vi "Brute Force Dark Current Primary Logic Body.vi"(0 "Data Pin in":refnum<k21>, 1 "Barcodes in":string[](array[string]), 2 "Sync Pin in":refnum<k21>, 3 "Channel #":i32, 4 "Write Pin in":refnum<k21>, 6 "Clear Pin in":refnum<k21>, 10 "Number of Tubes":i32, 14 "stop":bool) -> (8 "Actual Current Limit (nA)":dbl format="%#_13g", 15 "Mesurnment Itteration":i32, 16 "Power Supply Trip":bool, 20 "Data Pin out":refnum<k21>, 21 "Actual Voltage Level (V)":dbl format="%#_13g", 22 "Sync Pin out":refnum<k21>, 24 "Write Pin out":refnum<k21>, 26 "Clear Pin out":refnum<k21>)   [LabVIEW 2020]
panel:
  out "Manual Measurments \nNeeded":bool
  in  "VISA Refnum in":refnum<visa-resource-name>
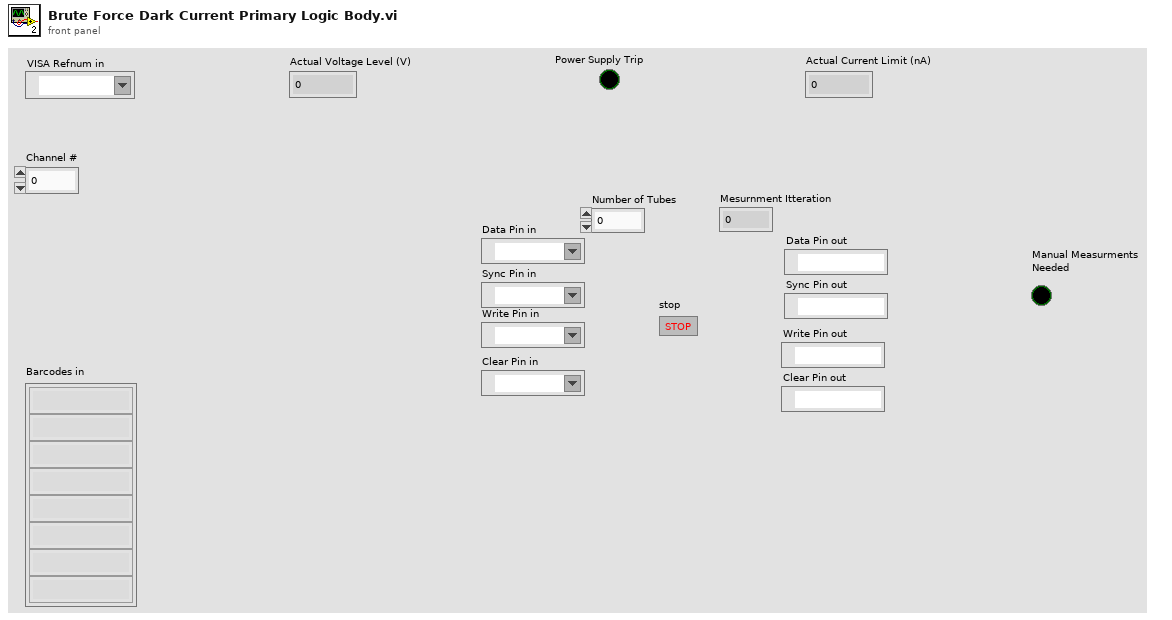
[diagram p1: front panel]
types:
  T1 = cluster{"VISA resource name":refnum<visa-resource-name>, "Board address":u8, "NChannels":u8}
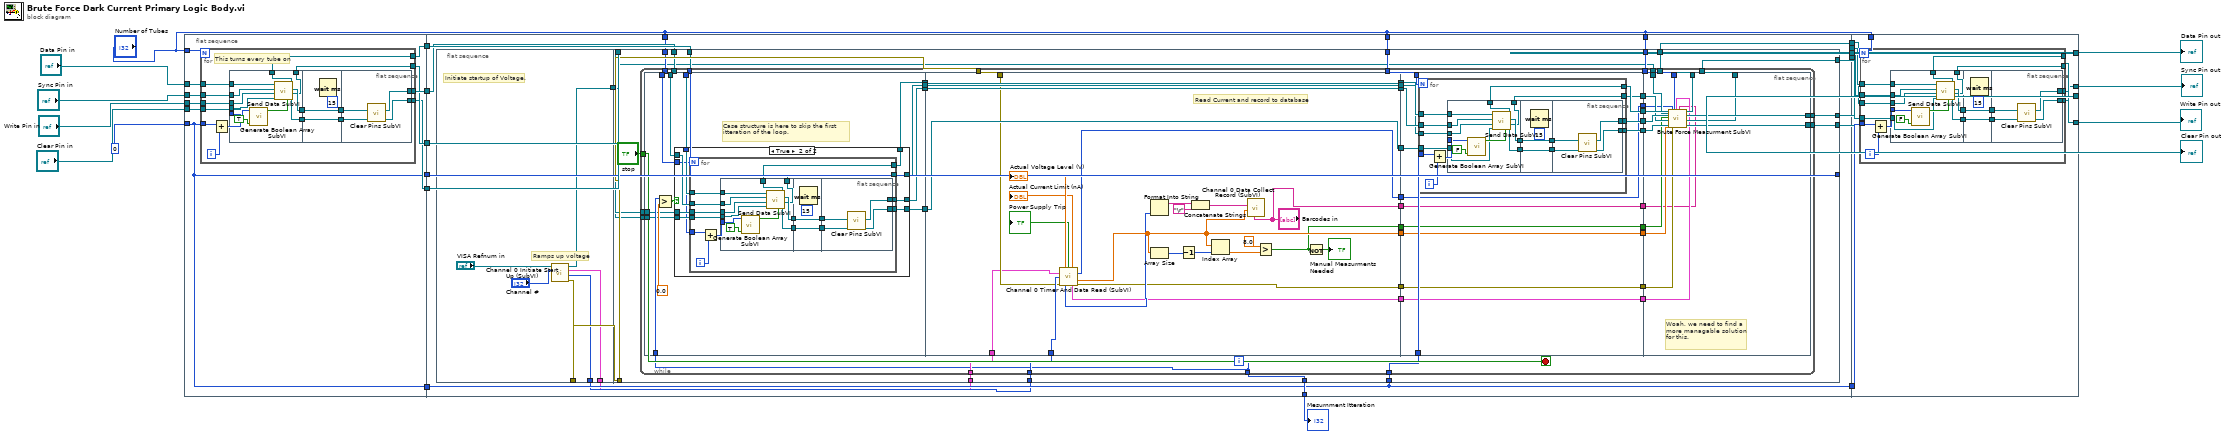
[diagram p0: block diagram]
diagram:
  n1 = flat-sequence {
    tunnel: 0 ("First Tube #") -> [w23]
    tunnel: "Number of Tubes" -> [w29]
    tunnel: "Data Pin in" -> [w32]
    tunnel: "Sync Pin in" -> [w31]
    tunnel: "Write Pin in" -> [w30]
    tunnel: [w23] -> w22
    tunnel: "Clear Pin in" -> [w28]
    tunnel: [w27] -> w6
    tunnel: [w26] -> w5
    tunnel: [w25] -> w4
    tunnel: [w24] -> w3
    tunnel: [w23] -> w1
    tunnel: w22 -> [w77]
    tunnel: [w77] -> w21
    tunnel: [w81] -> w20
    tunnel: [w80] -> w19
    tunnel: [w82] -> w18
    tunnel: [w79] -> w17
    tunnel: "Number of Tubes" -> [w83]
    tunnel: [w78] -> w7
    tunnel: w6 -> [w72]
    tunnel: w5 -> [w71]
    tunnel: w4 -> [w70]
    tunnel: w3 -> [w69]
    tunnel: "Number of Tubes" -> [w76]
    tunnel: "Number of Tubes" -> [w68]
    tunnel: w1 -> [w67]
    tunnel: w21 -> [w311]
    tunnel: w20 -> [w310]
    tunnel: w19 -> [w309]
    tunnel: w18 -> [w308]
    tunnel: w17 -> [w307]
    tunnel: [w306] -> w12
    tunnel: [w305] -> w11
    tunnel: [w304] -> w10
    tunnel: [w303] -> w9
    tunnel: "Number of Tubes" -> [w302]
    frame #0 {
      n2 = for {
        N: w29 -> [_]
        tunnel: w32 -> [w47]
        tunnel: w31 -> [w46]
        tunnel: w30 -> [w45]
        tunnel: [w44] -> w26
        tunnel: [w43] -> w24
        tunnel: [w42] -> w25
        tunnel: [w41] -> w27
        tunnel: w23 -> [w38]
        tunnel: w28 -> [w37]
        i -> [w39]
        # "This turns every tube on"
        n3 = Add(x=w38, y=w39) -> (x+y=w40:i32)
        n4 = flat-sequence {
          tunnel: w40 -> [w56]
          tunnel: w47 -> [w55]
          tunnel: w46 -> [w54]
          tunnel: w45 -> [w53]
          tunnel: [w52] -> w36
          tunnel: [w51] -> w34
          tunnel: [w50] -> w42
          tunnel: [w49] -> w41
          tunnel: w37 -> [w48]
          tunnel: w36 -> [w61]
          tunnel: [w61] -> w35
          tunnel: w34 -> [w60]
          tunnel: [w60] -> w33
          tunnel: w35 -> [w65]
          tunnel: w33 -> [w64]
          tunnel: [w63] -> w44
          tunnel: [w62] -> w43
          frame #0 {
            n5 = call "Generate Boolean Array SubVI.vi"("Activate: 1\nDeactivate: 0"=TRUE, "Tube"=w56) -> ("Boolean array"=w57:bool[])  [unwired: 9 in]
            n6 = call "Send Data SubVI.vi"("Data Pin Task In"=w55, "Sync Pin Task In"=w54, "Write Pin Task In"=w53, "Clear Pin Task In"=w48, "Data"=w57) -> ("Data Pin Task Out"=w49:refnum<k21>, "Sync Pin Task Out"=w52:refnum<k21>, "Write Pin Task Out"=w50:refnum<k21>, "Clear Pin Task Out"=w51:refnum<k21>)  [unwired: 1 in]
          }
          frame #1 {
            n7 = Wait (ms)(milliseconds to wait=u32 15) -> ()  [unwired: 1 out]
          }
          frame #2 {
            n8 = call "Clear Pins SubVI.vi"("Clear Pin Task In"=w64, "Sync Pin Task In"=w65) -> ("Clear Pin Task Out"=w62:refnum<k21>, "Sync Pin Task Out"=w63:refnum<k21>)  [unwired: 8 in]
          }
        }
      }
    }
    frame #1 {
      n9 = flat-sequence {
        tunnel: [w87] -> w74
        tunnel: [w86] -> w75
        tunnel: [w85] -> w73
        tunnel: [w84] -> w66
        tunnel: w83 -> [w107]
        tunnel: [w106] -> w82
        tunnel: [w105] -> w81
        tunnel: [w104] -> w80
        tunnel: [w103] -> w79
        tunnel: [w102] -> w78
        tunnel: w77 -> [w101]
        tunnel: w76 -> [w100]
        tunnel: w75 -> [w99]
        tunnel: w74 -> [w98]
        tunnel: w73 -> [w97]
        tunnel: w72 -> [w96]
        tunnel: w71 -> [w95]
        tunnel: w70 -> [w94]
        tunnel: w69 -> [w93]
        tunnel: w68 -> [w92]
        tunnel: w67 -> [w91]
        tunnel: w66 -> [w90]
        frame #0 {
          # "Ramps up voltage"
          # "Initiate startup of Voltage."
          n10 = call "Channel 0 Initiate Start Up (SubVI).vi"("Channel # in"="Channel #", "VISA Refnum in"="VISA Refnum in") -> ("error out"=w87:errorcluster, "Channel # out"=w86:i32, "BoardHandle out"=w85:T1, "VISA Refnum out"=w84:refnum<visa-resource-name>)  [unwired: 6 in]
        }
        frame #1 {
          n11 = while {
            tunnel: "stop" -> [w151]
            tunnel: w107 -> [w150]
            tunnel: [w149] -> w106
            tunnel: [w148] -> w105
            tunnel: [w147] -> w104
            tunnel: [w146] -> w103
            tunnel: [w136] -> w102
            tunnel: w101 -> [w141]
            tunnel: w100 -> [w140]
            tunnel: w99 -> [w139]
            tunnel: w98 -> [w138]
            tunnel: w97 -> [w137]
            tunnel: w96 -> [w135]
            tunnel: w95 -> [w134]
            tunnel: w94 -> [w133]
            tunnel: w93 -> [w132]
            tunnel: w92 -> [w123]
            tunnel: w91 -> [w122]
            tunnel: w90 -> [w115]
            i -> [w136]
            stop <- w151 stop-if-true
            n12 = flat-sequence {
              tunnel: w136 -> [w162]
              tunnel: w135 -> [w161]
              tunnel: w134 -> [w160]
              tunnel: w133 -> [w159]
              tunnel: w132 -> [w158]
              tunnel: [w157] -> w130
              tunnel: [w156] -> w128
              tunnel: [w155] -> w126
              tunnel: [w154] -> w124
              tunnel: w123 -> [w153]
              tunnel: w122 -> [w152]
              tunnel: w139 -> [w224]
              tunnel: w138 -> [w213]
              tunnel: w137 -> [w212]
              tunnel: [w223] -> w131
              tunnel: w130 -> [w223]
              tunnel: [w222] -> w129
              tunnel: w128 -> [w222]
              tunnel: [w221] -> w127
              tunnel: w126 -> [w221]
              tunnel: [w220] -> w125
              tunnel: w124 -> [w220]
              tunnel: [w219] -> w121
              tunnel: [w218] -> w118
              tunnel: [w217] -> w117
              tunnel: [w216] -> w113
              tunnel: [w215] -> w111
              tunnel: ["Barcodes in"] -> w109
              tunnel: [w252] -> w145
              tunnel: [w251] -> w144
              tunnel: [w250] -> w143
              tunnel: [w249] -> w142
              tunnel: w141 -> [w248]
              tunnel: w140 -> [w247]
              tunnel: w131 -> [w246]
              tunnel: w129 -> [w245]
              tunnel: w127 -> [w244]
              tunnel: w125 -> [w243]
              tunnel: w121 -> [w242]
              tunnel: [w242] -> w120
              tunnel: [w241] -> w119
              tunnel: w118 -> [w241]
              tunnel: w117 -> [w240]
              tunnel: [w240] -> w116
              tunnel: [w239] -> w114
              tunnel: w113 -> [w239]
              tunnel: [w238] -> w112
              tunnel: w111 -> [w238]
              tunnel: [w237] -> w110
              tunnel: w109 -> [w237]
              tunnel: w150 -> [w293]
              tunnel: [w301] -> w149
              tunnel: [w300] -> w148
              tunnel: [w299] -> w147
              tunnel: [w298] -> w146
              tunnel: w145 -> [w297]
              tunnel: w144 -> [w296]
              tunnel: w143 -> [w295]
              tunnel: w142 -> [w294]
              tunnel: w120 -> [w292]
              tunnel: w119 -> [w291]
              tunnel: w116 -> [w290]
              tunnel: w115 -> [w289]
              tunnel: w114 -> [w288]
              tunnel: w112 -> [w287]
              tunnel: w110 -> [w286]
              frame #0 {
                # "Case structure is here to skip the first itteration of the loop."
                n13 = Greater?(x=w162, y=0.0) -> (0:w164:bool)
                n14 = case shown="True" w164 {
                  tunnel: w161 -> [w168 w178]
                  tunnel: w160 -> [w167 w177]
                  tunnel: w159 -> [w166 w176]
                  tunnel: w158 -> [w165 w175]
                  tunnel: [w168 w174] -> w157
                  tunnel: [w167 w173] -> w156
                  tunnel: [w166 w172] -> w155
                  tunnel: [w165 w171] -> w154
                  tunnel: w153 -> [_ w170]
                  tunnel: w152 -> [_ w169]
                  frame False {
                  }
                  frame True {
                    n15 = for {
                      N: w170 -> [_]
                      tunnel: w178 -> [w193]
                      tunnel: w177 -> [w192]
                      tunnel: w176 -> [w191]
                      tunnel: [w190] -> w173
                      tunnel: [w189] -> w171
                      tunnel: [w188] -> w172
                      tunnel: [w187] -> w174
                      tunnel: w169 -> [w184]
                      tunnel: w175 -> [w183]
                      i -> [w185]
                      n16 = Add(x=w184, y=w185) -> (x+y=w186:i32)
                      n17 = flat-sequence {
                        tunnel: w186 -> [w202]
                        tunnel: w193 -> [w201]
                        tunnel: w192 -> [w200]
                        tunnel: w191 -> [w199]
                        tunnel: [w198] -> w182
                        tunnel: [w197] -> w180
                        tunnel: [w196] -> w188
                        tunnel: [w195] -> w187
                        tunnel: w183 -> [w194]
                        tunnel: w182 -> [w207]
                        tunnel: [w207] -> w181
                        tunnel: w180 -> [w206]
                        tunnel: [w206] -> w179
                        tunnel: w181 -> [w211]
                        tunnel: w179 -> [w210]
                        tunnel: [w209] -> w190
                        tunnel: [w208] -> w189
                        frame #0 {
                          n18 = call "Generate Boolean Array SubVI.vi"("Activate: 1\nDeactivate: 0"=TRUE, "Tube"=w202) -> ("Boolean array"=w203:bool[])  [unwired: 9 in]
                          n19 = call "Send Data SubVI.vi"("Data Pin Task In"=w201, "Sync Pin Task In"=w200, "Write Pin Task In"=w199, "Clear Pin Task In"=w194, "Data"=w203) -> ("Data Pin Task Out"=w195:refnum<k21>, "Sync Pin Task Out"=w198:refnum<k21>, "Write Pin Task Out"=w196:refnum<k21>, "Clear Pin Task Out"=w197:refnum<k21>)  [unwired: 1 in]
                        }
                        frame #1 {
                          n20 = Wait (ms)(milliseconds to wait=u32 15) -> ()  [unwired: 1 out]
                        }
                        frame #2 {
                          n21 = call "Clear Pins SubVI.vi"("Clear Pin Task In"=w210, "Sync Pin Task In"=w211) -> ("Clear Pin Task Out"=w208:refnum<k21>, "Sync Pin Task Out"=w209:refnum<k21>)  [unwired: 8 in]
                        }
                      }
                    }
                  }
                }
              }
              frame #1 {
                # "Read Current and record to database"
                n22 = call "Channel 0 Timer And Data Read (SubVI).vi"("BoardHandle in"=w212, "Channel # in"=w224, "error in (no error)"=w213) -> ("Actual Voltage Level (V)"=→"Actual Voltage Level (V)":dbl, "Power Supply Trip"=→"Power Supply Trip":bool, "Actual Current Limit (nA)"=→"Actual Current Limit (nA)":dbl, "Channel # out 2"=w216:i32, "Array"=w218:dbl[], "dt (s) out"=w232:i32, "BoardHandle out 2"=w215:T1, "error out"=w219:errorcluster)  [unwired: 5 in]
                n23 = Format Into String(w232) -> (resulting string=w230:string)  [unwired: 3 in, 1 out]
                n24 = Array Size(array=w218) -> (size(s)=w236:i32)
                n25 = Decrement(x=w236) -> (x-1=w235:i32)
                n26 = Concatenate Strings(w230, "\r") -> (w231:string)
                n27 = Index Array(array=w218, index=w235) -> (element=w234:dbl)
                n28 = call "Channel 0 Data Collect Record (SubVI).vi"("Barcodes"="Barcodes in", "Array"=w218, "String"=w231) -> ()  [unwired: 9 in]
                n29 = Greater?(x=8.0, y=w234) -> (0:w217:bool)
                n30 = Not(x=w217) -> (.not. x?=→"Manual Measurments \nNeeded":bool)
              }
              frame #2 {
                n31 = for {
                  N: w247 -> [_]
                  tunnel: w246 -> [w267]
                  tunnel: w245 -> [w266]
                  tunnel: w244 -> [w265]
                  tunnel: [w264] -> w251
                  tunnel: [w263] -> w249
                  tunnel: [w262] -> w250
                  tunnel: [w261] -> w252
                  tunnel: w248 -> [w258]
                  tunnel: w243 -> [w257]
                  i -> [w259]
                  n32 = Add(x=w258, y=w259) -> (x+y=w260:i32)
                  n33 = flat-sequence {
                    tunnel: w260 -> [w276]
                    tunnel: w267 -> [w275]
                    tunnel: w266 -> [w274]
                    tunnel: w265 -> [w273]
                    tunnel: [w272] -> w256
                    tunnel: [w271] -> w254
                    tunnel: [w270] -> w262
                    tunnel: [w269] -> w261
                    tunnel: w257 -> [w268]
                    tunnel: w256 -> [w281]
                    tunnel: [w281] -> w255
                    tunnel: w254 -> [w280]
                    tunnel: [w280] -> w253
                    tunnel: w255 -> [w285]
                    tunnel: w253 -> [w284]
                    tunnel: [w283] -> w264
                    tunnel: [w282] -> w263
                    frame #0 {
                      n34 = call "Generate Boolean Array SubVI.vi"("Activate: 1\nDeactivate: 0"=FALSE, "Tube"=w276) -> ("Boolean array"=w277:bool[])  [unwired: 9 in]
                      n35 = call "Send Data SubVI.vi"("Data Pin Task In"=w275, "Sync Pin Task In"=w274, "Write Pin Task In"=w273, "Clear Pin Task In"=w268, "Data"=w277) -> ("Data Pin Task Out"=w269:refnum<k21>, "Sync Pin Task Out"=w272:refnum<k21>, "Write Pin Task Out"=w270:refnum<k21>, "Clear Pin Task Out"=w271:refnum<k21>)  [unwired: 1 in]
                    }
                    frame #1 {
                      n36 = Wait (ms)(milliseconds to wait=u32 15) -> ()  [unwired: 1 out]
                    }
                    frame #2 {
                      n37 = call "Clear Pins SubVI.vi"("Clear Pin Task In"=w284, "Sync Pin Task In"=w285) -> ("Clear Pin Task Out"=w282:refnum<k21>, "Sync Pin Task Out"=w283:refnum<k21>)  [unwired: 8 in]
                    }
                  }
                }
              }
              frame #3 {
                # "Woah, we need to find a more managable solution for this."
                n38 = call "Brute Force Measurment SubVI.vi"("Data Pin Task In"=w297, "VISA Refnum in"=w289, "Sync Pin Task In"=w296, "Boolean 9"=w290, "Write Pin Task In"=w295, "Clear Pin Task In"=w294, "Array"=w291, "Channel # in"=w288, "error in (no error)"=w292, "Number of Active tubes"=w293, "BoardHandle in"=w287, "Barcodes in"=w286) -> ("Data Pin Task Out"=w301:refnum<k21>, "Sync Pin Task Out"=w300:refnum<k21>, "Write Pin Task Out"=w299:refnum<k21>, "Clear Pin Task Out"=w298:refnum<k21>)  [unwired: 12 in]
              }
            }
          }
        }
      }
    }
    frame #2 {
      n39 = for {
        N: w302 -> [_]
        tunnel: w310 -> [w326]
        tunnel: w309 -> [w325]
        tunnel: w308 -> [w324]
        tunnel: [w323] -> w304
        tunnel: [w322] -> w303
        tunnel: [w321] -> w305
        tunnel: [w320] -> w306
        tunnel: w311 -> [w317]
        tunnel: w307 -> [w316]
        i -> [w318]
        n40 = Add(x=w317, y=w318) -> (x+y=w319:i32)
        n41 = flat-sequence {
          tunnel: w319 -> [w335]
          tunnel: w326 -> [w334]
          tunnel: w325 -> [w333]
          tunnel: w324 -> [w332]
          tunnel: [w331] -> w315
          tunnel: [w330] -> w313
          tunnel: [w329] -> w321
          tunnel: [w328] -> w320
          tunnel: w316 -> [w327]
          tunnel: w315 -> [w340]
          tunnel: [w340] -> w314
          tunnel: w313 -> [w339]
          tunnel: [w339] -> w312
          tunnel: w314 -> [w344]
          tunnel: w312 -> [w343]
          tunnel: [w342] -> w323
          tunnel: [w341] -> w322
          frame #0 {
            n42 = call "Generate Boolean Array SubVI.vi"("Activate: 1\nDeactivate: 0"=FALSE, "Tube"=w335) -> ("Boolean array"=w336:bool[])  [unwired: 9 in]
            n43 = call "Send Data SubVI.vi"("Data Pin Task In"=w334, "Sync Pin Task In"=w333, "Write Pin Task In"=w332, "Clear Pin Task In"=w327, "Data"=w336) -> ("Data Pin Task Out"=w328:refnum<k21>, "Sync Pin Task Out"=w331:refnum<k21>, "Write Pin Task Out"=w329:refnum<k21>, "Clear Pin Task Out"=w330:refnum<k21>)  [unwired: 1 in]
          }
          frame #1 {
            n44 = Wait (ms)(milliseconds to wait=u32 15) -> ()  [unwired: 1 out]
          }
          frame #2 {
            n45 = call "Clear Pins SubVI.vi"("Clear Pin Task In"=w343, "Sync Pin Task In"=w344) -> ("Clear Pin Task Out"=w341:refnum<k21>, "Sync Pin Task Out"=w342:refnum<k21>)  [unwired: 8 in]
          }
        }
      }
    }
  }
  "Data Pin out" <- w12
  "Sync Pin out" <- w10
  "Write Pin out" <- w11
  "Clear Pin out" <- w9
  "Mesurnment Itteration" <- w7
